vi "Run.vi"(8 "error in (no error)":errorcluster caption="entrée d'erreur (pas d'erreur)", 10 "X":string[][](array[string]), 11 "power_transform.lvclass":refnum<class "power_transform.lvclass">) -> (0 "error out":errorcluster caption="sortie d'erreur", 2 "Data":T1, 3 "power_transform.lvclass":refnum<class "power_transform.lvclass">)   [LabVIEW 2020, in "power_transform.lvclass"]
doc: "Returns : \n\n- X_trans : array-like, shape (n_samples, n_features)\nThe transformed data."
uses:
  power_transform.lvclass
  power_transform.lvclass/power_transform.ctl
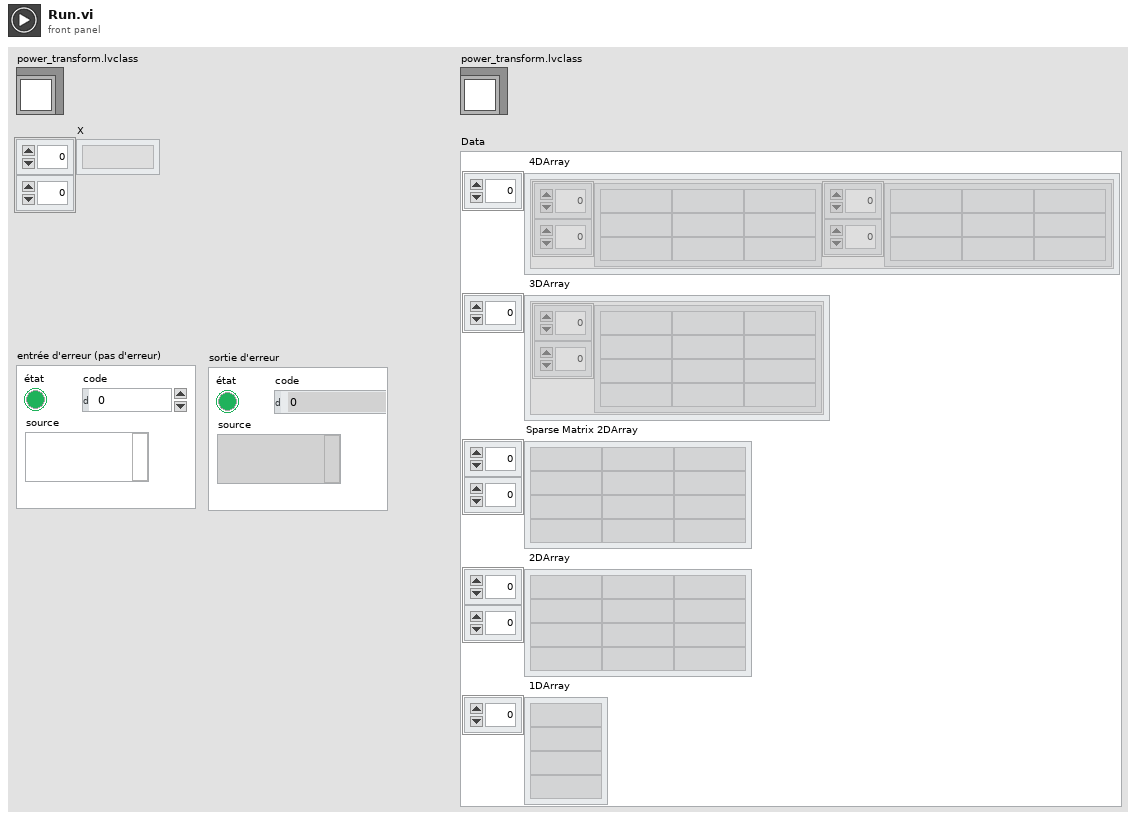
[diagram p1: front panel]
types:
  T1 = cluster{" 4DArray":cluster{"1":string[][], "2":string[][]}[], " 3DArray":cluster{"Tableau":string[][]}[], "Sparse Matrix 2DArray":string[][], " 2DArray":string[][], " 1DArray":string[]}
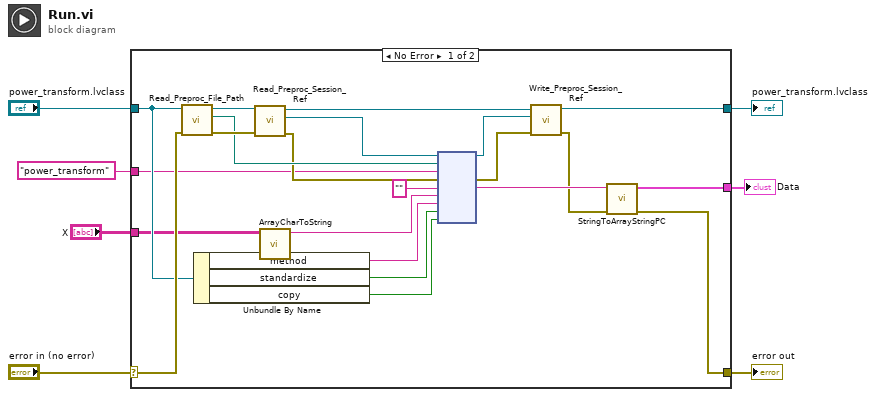
[diagram p0: block diagram]
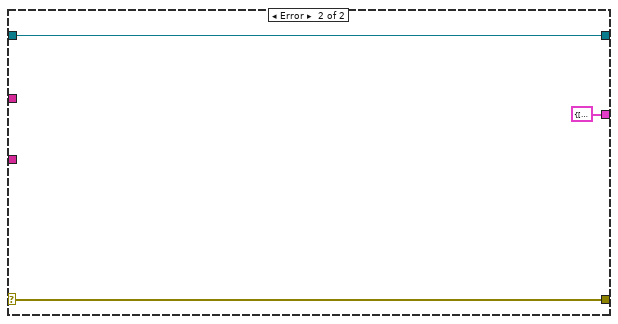
[diagram p2: hidden frame]
diagram:
  n1 = case shown="No Error" "error in (no error)" {
    selector: "error in (no error)" -> [w18 w32]
    tunnel: [w8 w32] -> w6
    tunnel: [w9 w31] -> w4
    tunnel: "power_transform.lvclass" -> [w17 w31]
    tunnel: [w10 T1 {" 4DArray"=[], " 3DArray"=[], "Sparse Matrix 2DArray"=[], " 2DArray"=[], " 1DArray"=[]} ("Data")] -> w3
    tunnel: "power_transform" ("Fonction") -> [w16 _]
    tunnel: "X" -> [w14 _]
    frame No Error {
      n2 = call-dynamic "Read_Preproc_File_Path.vi"("error in (no error)"=w18, "Python in"=w17) -> ("error out"=w28:errorcluster, "File_Path"=w25:path, "Python out"=w29:refnum<class "power_transform.lvclass">)  [unwired: 7 in]
      n3 = Unbundle By Name(w17) -> ("method"=w20:string, "standardize"=w19:bool, "copy"=w15:bool)
      n4 = call-dynamic "Read_Preproc_Session_Ref.vi"("error in (no error)"=w28, "Python in"=w29) -> ("error out"=w24:errorcluster, "Session_ref"=w26:refnum<k35>, "Python out"=w27:refnum<class "power_transform.lvclass">)  [unwired: 7 in]
      n5 = call "ArrayCharToString.vi"("TAB"=w14) -> ("Instruction"=w13:string)  [unwired: 10 in]
      n6 = node(w26, w25, w16, w24, "", w13, w20, w19, w15) -> (w22:refnum<k35>, w23:errorcluster, w12:string)  [unwired: 4 in, 2 out]
      n7 = call-dynamic "Write_Preproc_Session_Ref.vi"("error in (no error)"=w23, "Session_ref"=w22, "Python in"=w27) -> ("error out"=w11:errorcluster, "Python out"=w9:refnum<class "power_transform.lvclass">)  [unwired: 7 in]
      n8 = call "StringToArrayStringPC.vi"("sortie d'erreur"=w11, "Return value"=w12) -> ("sortie d'erreur"=w8:errorcluster, "Data"=w10:T1)  [unwired: 8 in]
    }
    frame Error {
    }
  }
  "error out" <- w6
  "power_transform.lvclass" <- w4
  "Data" <- w3
